vi "MWC Global.vi"() -> ()   [LabVIEW 2019]
panel:
  in  "HP Device":string
  in  "Tune Time Unit":i32
  in  "Switch MSB Chan":i32
  in  "Switch LSB Chan":i32
  in  "Tune Down Chan":i32
  in  "Tune Up Chan":i32
  in  "DIO Device":i32
  in  "FM Device":string
  in  "Bellows Device":string
  in  "EIP Device":string
  in  "Power Meter Channel":i32=7
  in  "Power Meter Device":i32=1
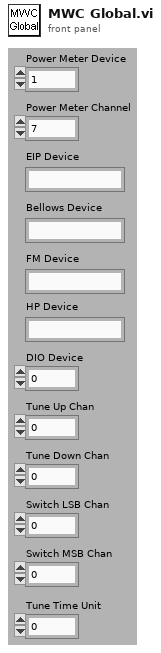
[diagram p1: front panel]
diagram:
